vi "Write.vi"(8 "error in (no error)":errorcluster, 9 "Data":u8[](array[numeric]), 10 "I2C Slave Address":u8, 11 "I2C in":refnum<class "I2C.lvclass">) -> (0 "error out":errorcluster, 3 "I2C out":refnum<class "I2C.lvclass">)   [LabVIEW 2014, in "I2C.lvclass"]
doc: "Write data bytes to the I2C slave device identified by I2C Slave Address."
uses:
  I2C.lvclass
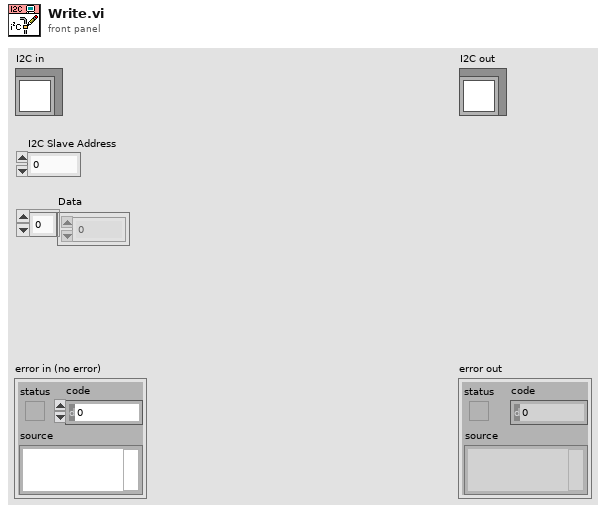
[diagram p1: front panel]
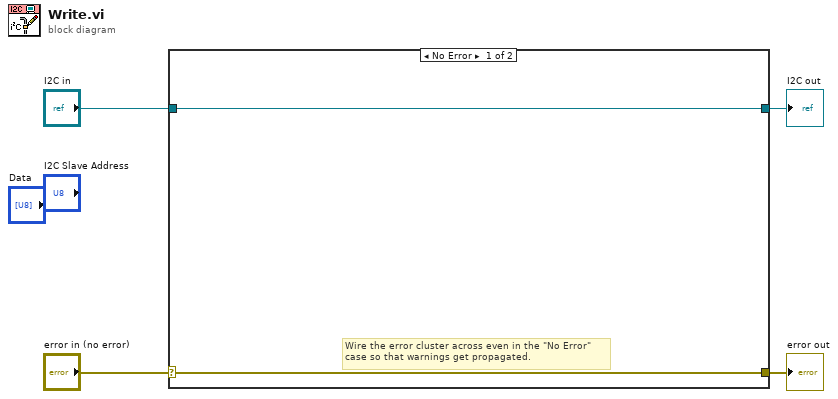
[diagram p0: block diagram]
diagram:
  n1 = case shown="No Error" "error in (no error)" {
    selector: "error in (no error)" -> [w5 w8]
    tunnel: [w5 w8] -> w3
    tunnel: [w6 w7] -> w1
    tunnel: "I2C in" -> [w6 w7]
    frame No Error {
      # "Wire the error cluster across even in the \"No Error\"\ncase so that warnings get propagated."
    }
    frame Error {
    }
  }
  "error out" <- w3
  "I2C out" <- w1
